vi "Write Config info.vi"(10 "Config info":T1={"RBW"=0.0, "VBW "=0.0, "Number of Averages"=0, "Average On"=FALSE, "Symbols"=[], "All Harm"=FALSE, "Loop order"=enum."Device -> Power -> Frequency", "Power Window"=0.0, "Frequency (MHz)"="900", "Power (dBm)"="-40:-30/2", "PM for power leveling"=0, "Zero span"=FALSE, "Stop level"=999.0}, 11 "Harmonics in":refnum<class "Harmonics.lvclass">) -> (3 "Harmonics out":refnum<class "Harmonics.lvclass">)   [LabVIEW 2020, in "Harmonics.lvclass"]
uses:
  Harmonics.lvclass
  Controls/Config info.ctl
  Controls/Loop order.ctl
  Harmonics.lvclass/Harmonics.ctl
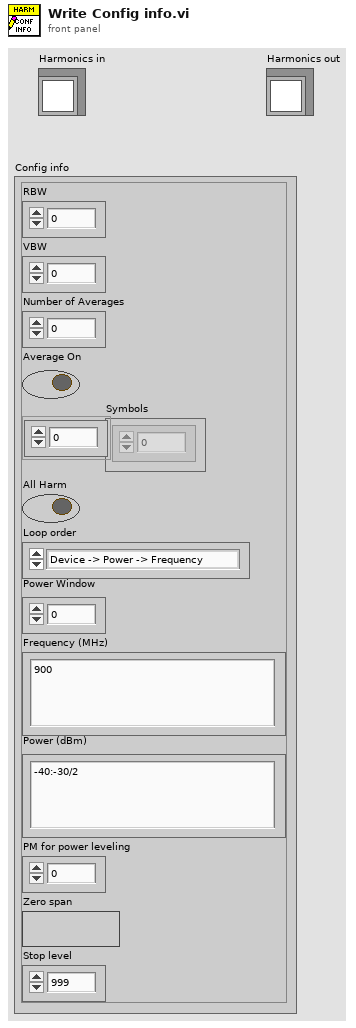
[diagram p1: front panel]
types:
  T1 = typedef "Harmonics.lvclass/Config info.ctl" = cluster{"RBW":dbl, "VBW ":dbl, "Number of Averages":i32, "Average On":bool, "Symbols":i32[], "All Harm":bool, "Loop order":T2, "Power Window":dbl, "Frequency (MHz)":string, "Power (dBm)":string, "PM for power leveling":u8, "Zero span":bool, "Stop level":dbl}
  T2 = typedef "Harmonics.lvclass/Loop order.ctl" = enum16{"Device -> Power -> Frequency", "Device -> Frequency -> Power"}
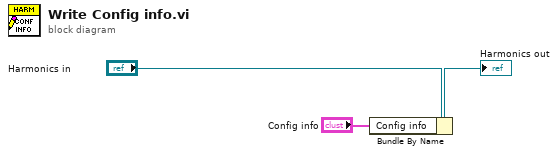
[diagram p0: block diagram]
diagram:
  n1 = Bundle By Name(cluster="Harmonics in", "Config info"="Config info") -> (→"Harmonics out":refnum<class "Harmonics.lvclass">)
